vi "Update Active Chassis.vi"(8 "error in (no error)":errorcluster, 10 "Active Chassis":string, 11 "FP Controls in":refnum<class "FP Controls.lvclass">) -> (0 "error out":errorcluster, 3 "FP Controls out":refnum<class "FP Controls.lvclass">)   [LabVIEW 2018, in "Configuration Grandmaster.lvlib" / "FP Controls.lvclass"]
uses:
  FP Controls.lvclass
  FP Controls.lvclass/FP Controls.ctl
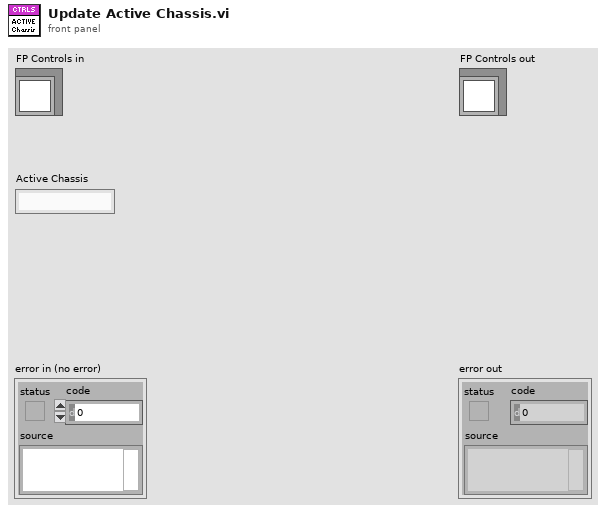
[diagram p1: front panel]
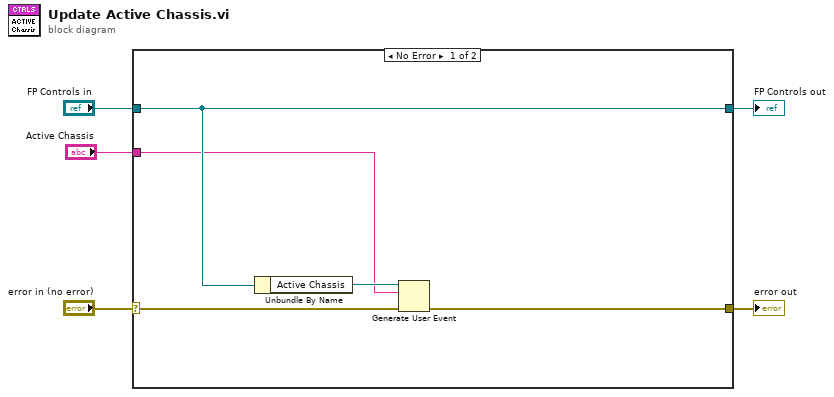
[diagram p0: block diagram]
diagram:
  n1 = case shown="No Error" "error in (no error)" {
    selector: "error in (no error)" -> [w10 w12]
    tunnel: [w9 w12] -> w4
    tunnel: [w8 w11] -> w2
    tunnel: "FP Controls in" -> [w8 w11]
    tunnel: "Active Chassis" -> [w6 _]
    frame No Error {
      n2 = Unbundle By Name(w8) -> ("Active Chassis"=w7:refnum<user-event>)
      n3 = Generate User Event(user event=w7, event data cluster=w6, error in=w10) -> (error out=w9:errorcluster)  [unwired: 1 in, 1 out]
    }
    frame Error {
    }
  }
  "error out" <- w4
  "FP Controls out" <- w2
